vi "obs_avoid.vi"(11 "shifthold":dbl=0.02) -> (3 "obs shift":dbl format="%.2f")   [LabVIEW 2015]
uses:
  G_ALL.vi
  G_SEN.vi
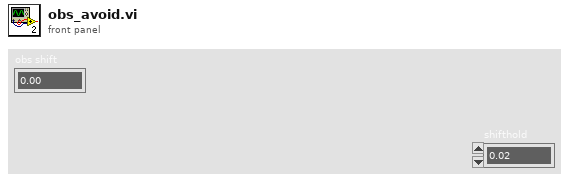
[diagram p1: front panel]
types:
  T1 = cluster{"Steer_input":dbl, "Steer_output":dbl, "VS_des":dbl, "VS_can":dbl, "heading":dbl, "auto":bool, "run":bool, "x":dbl, "y":dbl}
  T2 = cluster{"C_Wheel base":dbl, "ratio_steer":dbl, "Overall width":dbl, "af":dbl, "turn radius":dbl, "eval":dbl, "ap":dbl, "an":dbl, "Vmax":dbl, "mu":dbl, "Vlast":dbl}
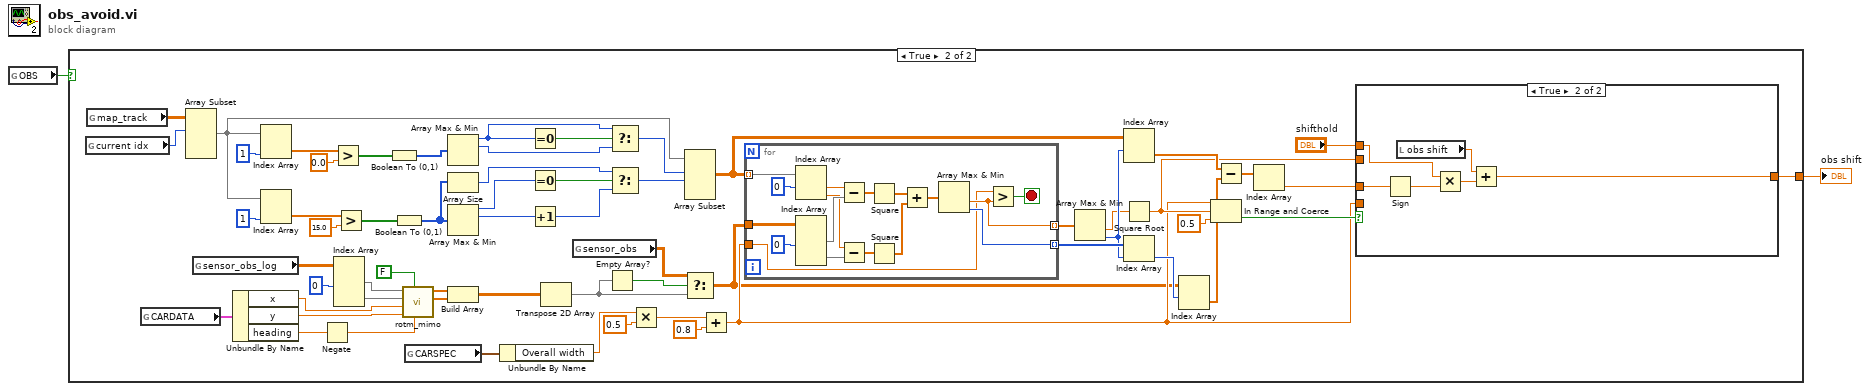
[diagram p0: block diagram]
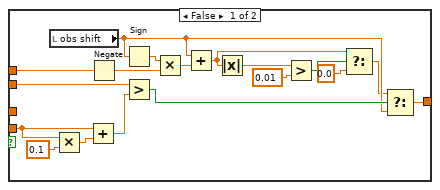
[diagram p3: hidden frame]
diagram:
  n1 = global read "G_ALL.vi" "OBS"() -> (w1:bool)
  n2 = case shown="True" w1 {
    tunnel: [_ w51] -> w2
    frame False {
    }
    frame True {
      n3 = global read "G_ALL.vi" "current idx"() -> (w4:i32)
      n4 = global read "G_ALL.vi" "map_track"() -> (w5:dbl[][])
      n5 = global read "G_ALL.vi" "CARDATA"() -> (w33:T1)
      n6 = Array Subset(array=w5, index (row)=w4) -> (w3:dbl[][])  [unwired: 3 in]
      n7 = global read "G_SEN.vi" "sensor_obs_log"() -> (w37:dbl[][])
      n8 = Unbundle By Name(w33) -> ("x"=w41:dbl, "y"=w42:dbl, "heading"=w40:dbl)
      n9 = Index Array(array=w3, index (col)=1 ("disabled index (col)")) -> (element=w12:dbl[])  [unwired: 1 in]
      n10 = Index Array(array=w3, index (col)=1 ("disabled index (col)")) -> (element=w24:dbl[])  [unwired: 1 in]
      n11 = Negate(x=w40) -> (-x=w43:dbl)
      n12 = Greater?(x=w12, y=0.0) -> (0:w11:bool[])
      n13 = Index Array(array=w37, index (col) #1=0 ("disabled index (col)")) -> (element #1=w39:dbl[], element #2=w38:dbl[])  [unwired: 3 in]
      n14 = Greater?(x=w24, y=15.0) -> (0:w22:bool[])
      n15 = Boolean To (0,1)(Boolean=w11) -> (0, 1=w10:i16[])
      n16 = Boolean To (0,1)(Boolean=w22) -> (0, 1=w18:i16[])
      n17 = call "rotm_mimo.vi"("angle[rad]"=w43, "reverse"=FALSE, "y0"=w42, "x0"=w41, "y"=w38, "x"=w39) -> ("Y"=w35:dbl[], "X"=w36:dbl[])  [unwired: 2 in, 2 out]
      n18 = global read "G_ALL.vi" "CARSPEC"() -> (w32:T2)
      n19 = Array Max & Min(array=w10) -> (max value=w7:i16, max index (indices)=w8:i32)  [unwired: 2 out]
      n20 = Array Size(array=w18) -> (size(s)=w17:i32)
      n21 = Array Max & Min(array=w18) -> (max value=w21:i16, max index (indices)=w20:i32)  [unwired: 2 out]
      n22 = Build Array(w36, w35) -> (w34:dbl[][])
      n23 = Unbundle By Name(w32) -> ("Overall width"=w31:dbl)
      n24 = Equal To 0?(x=w7) -> (x = 0?=w9:bool)
      n25 = Equal To 0?(x=w21) -> (x = 0?=w19:bool)
      n26 = Increment(x=w20) -> (x+1=w16:i32)
      n27 = Transpose 2D Array(2D array=w34) -> (transposed array=w27:dbl[][])
      n28 = global read "G_SEN.vi" "sensor_obs"() -> (w29:dbl[][])
      n29 = Empty Array?(array=w27) -> (empty?=w30:bool)
      n30 = Select(t=w7, s=w9, f=w8) -> (s? t:f=w6:i32)
      n31 = Select(t=w17, s=w19, f=w16) -> (s? t:f=w15:i32)
      n32 = Multiply(x=w31, y=0.5) -> (x*y=w49:dbl)
      n33 = Array Subset(array=w3, index (row)=w6, length (row)=w15) -> (w26:dbl[][])  [unwired: 2 in]
      n34 = Select(t=w29, s=w30, f=w27) -> (s? t:f=w28:dbl[][])
      n35 = Add(x=w49, y=0.8) -> (x+y=w48:dbl)
      n36 = for {
        tunnel: w26 -> [w102] mode=indexing
        tunnel: w28 -> [w104]
        tunnel: [w90] -> w62 mode=indexing
        tunnel: [w91] -> w63 mode=indexing
        tunnel: w48 -> [w88]
        stop <- w89 stop-if-true
        n37 = Index Array(array=w102, index #1=0 ("index")) -> (element #1=w100:dbl, element #2=w98:dbl)  [unwired: 1 in]
        n38 = Index Array(array=w104, index (col) #1=0 ("disabled index (col)")) -> (element #1=w99:dbl[], element #2=w97:dbl[])  [unwired: 3 in]
        n39 = Subtract(x=w100, y=w99) -> (x-y=w96:dbl[])
        n40 = Subtract(x=w98, y=w97) -> (x-y=w95:dbl[])
        n41 = Square(x=w96) -> (x^2=w94:dbl[])
        n42 = Square(x=w95) -> (x^2=w93:dbl[])
        n43 = Add(x=w94, y=w93) -> (x+y=w92:dbl[])
        n44 = Array Max & Min(array=w92) -> (min value=w90:dbl, min index (indices)=w91:i32)  [unwired: 2 out]
        n45 = Greater?(x=w88, y=w90) -> (0:w89:bool)
      }
      n46 = Array Max & Min(array=w62) -> (min value=w56:dbl, min index (indices)=w60:i32)  [unwired: 2 out]
      n47 = Index Array(array=w26, index (row)=w60) -> (element=w59:dbl[])  [unwired: 1 in]
      n48 = Square Root(x=w56) -> (sqrt(x)=w52:dbl)
      n49 = Index Array(array=w63, index=w60) -> (element=w61:i32)
      n50 = Index Array(array=w28, index (row)=w61) -> (element=w58:dbl[])  [unwired: 1 in]
      n51 = In Range and Coerce(upper limit=w48, x=w52, lower limit=0.5) -> (In Range?=w54:bool)  [unwired: 1 out]
      n52 = Subtract(x=w59, y=w58) -> (x-y=w57:dbl[])
      n53 = Index Array(array=w57) -> (element=w53:dbl)  [unwired: 1 in]
      n54 = case shown="True" w54 {
        tunnel: w53 -> [_ w87]
        tunnel: [w79 w84] -> w51
        tunnel: w52 -> [w81 _]
        tunnel: "shifthold" -> [w65 w83]
        tunnel: w48 -> [w64 _]
        frame False {
          n55 = local read "obs shift"() -> (w76:dbl)
          n56 = Multiply(x=w64, y=0.1) -> (x*y=w68:dbl)
          n57 = Add(x=w64, y=w68) -> (x+y=w67:dbl)
          n58 = Negate(x=w65) -> (-x=w66:dbl)
          n59 = Sign(1:w76) -> (0:w78:dbl)
          n60 = Greater?(x=w81, y=w67) -> (0:w80:bool)
          n61 = Multiply(x=w78, y=w66) -> (x*y=w77:dbl)
          n62 = Add(x=w76, y=w77) -> (x+y=w72:dbl)
          n63 = Absolute Value(x=w72) -> (abs(x)=w75:dbl)
          n64 = Greater?(x=w75, y=0.01) -> (0:w73:bool)
          n65 = Select(t=w72, s=w73, f=0.0) -> (s? t:f=w70:dbl)
          n66 = Select(t=w70, s=w80, f=w76) -> (s? t:f=w79:dbl)
        }
        frame True {
          n67 = Sign(1:w87) -> (0:w82:dbl)
          n68 = local read "obs shift"() -> (w85:dbl)
          n69 = Multiply(x=w83, y=w82) -> (x*y=w86:dbl)
          n70 = Add(x=w85, y=w86) -> (x+y=w84:dbl)
        }
      }
    }
  }
  "obs shift" <- w2
